vi "Write config file path.vi"(8 "error in (no error)":errorcluster, 10 "config file path":path, 11 "_camera in":refnum<class "_camera.lvclass">) -> (0 "error out":errorcluster, 3 "_camera out":refnum<class "_camera.lvclass">)   [LabVIEW 2019, in "_camera.lvlib" / "_camera.lvclass"]
uses:
  _camera.lvclass
  _camera.lvclass/_camera.ctl
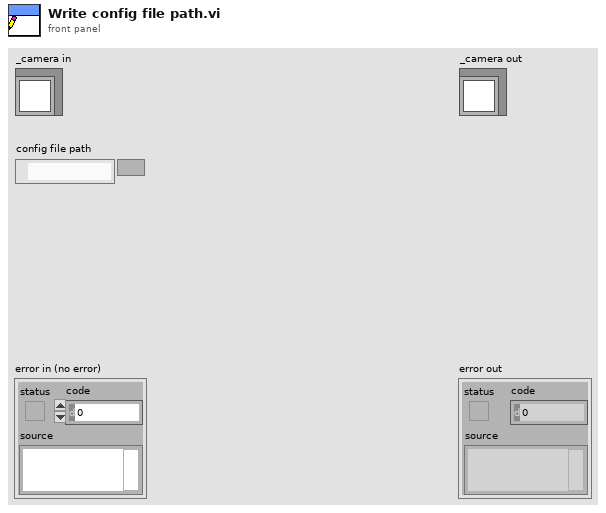
[diagram p1: front panel]
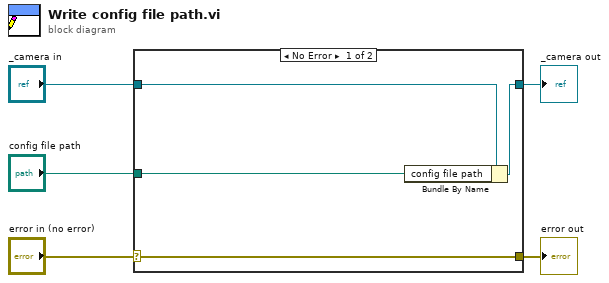
[diagram p0: block diagram]
diagram:
  n1 = case shown="No Error" "error in (no error)" {
    selector: "error in (no error)" -> [w9 w10]
    tunnel: [w9 w10] -> w4
    tunnel: [w7 w11] -> w2
    tunnel: "_camera in" -> [w8 w11]
    tunnel: "config file path" -> [w6 _]
    frame No Error {
      n2 = Bundle By Name(cluster=w8, "config file path"=w6) -> (w7:refnum<class "_camera.lvclass">)
    }
    frame Error {
    }
  }
  "error out" <- w4
  "_camera out" <- w2
